vi "updateTriggerList.vi"(8 "error in (no error)":errorcluster, 10 "Trigger list":T1(array[cluster]), 11 "Trigger queue in":refnum<queue>) -> (0 "error out":errorcluster, 1 "Trigger available?":bool, 2 "Updated trigger list":T1(array[cluster]), 3 "Trigger queue out":refnum<queue>)   [LabVIEW 2017]
uses:
  Trigger message.ctl
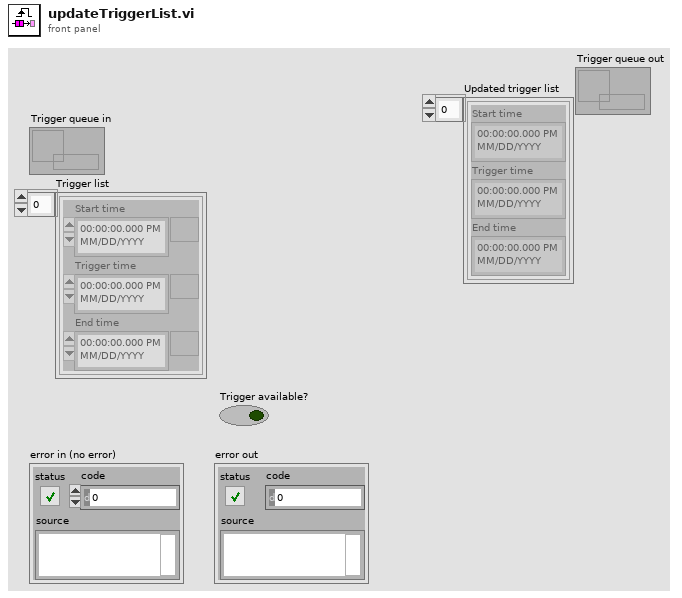
[diagram p1: front panel]
types:
  T1 = cluster{"Start time":timestamp, "Trigger time":timestamp, "End time":timestamp}[]
  T2 = typedef "Trigger message.ctl" = enum16{"New trigger", "Updated trigger"}
  T3 = cluster{"Trigger timestamps":cluster{"Start time":timestamp, "Trigger time":timestamp, "End time":timestamp}, "Message type":T2}
  T4 = cluster{"Start time":timestamp, "Trigger time":timestamp, "End time":timestamp}
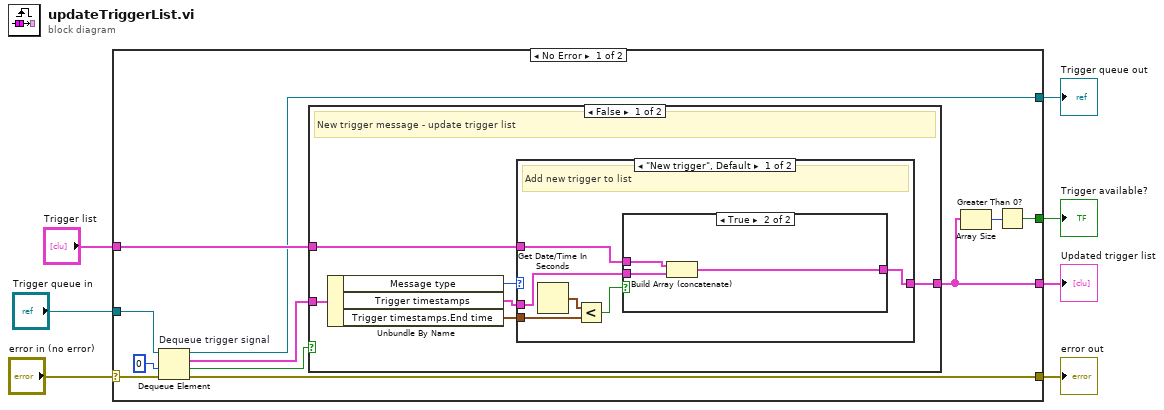
[diagram p0: block diagram]
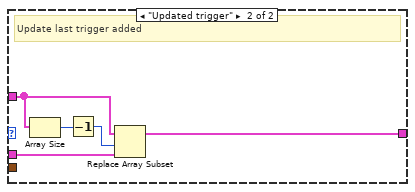
[diagram p3: hidden frame]
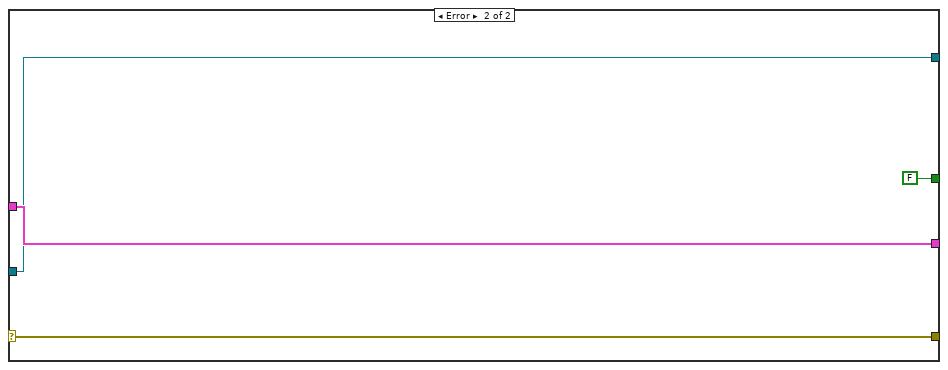
[diagram p5: hidden frame]
diagram:
  n1 = case shown="No Error" "error in (no error)" {
    selector: "error in (no error)" -> [w17 w44]
    tunnel: [w12 w44] -> w7
    tunnel: "Trigger queue in" -> [w16 w42]
    tunnel: "Trigger list" -> [w13 w43]
    tunnel: [w10 w43] -> w3
    tunnel: [w11 w42] -> w2
    tunnel: [w8 FALSE] -> w1
    frame No Error {
      n2 = Dequeue Element "Dequeue trigger signal"(queue=w16, timeout in ms (-1)=0, error in (no error)=w17) -> (queue out=w11:refnum<queue>, element=w14:T3, timed out?=w15:bool, error out=w12:errorcluster)
      n3 = case shown="False" w15 {
        tunnel: w14 -> [w23 _]
        tunnel: w13 -> [w24 w40]
        tunnel: [w20 w40] -> w10
        frame False {
          # "New trigger message - update trigger list"
          n4 = Unbundle By Name(w23) -> ("Message type"=w22:T2, "Trigger timestamps"=w21:T4, "Trigger timestamps.End time"=w19:timestamp)
          n5 = case shown="\"New trigger\", Default" w22 {
            tunnel: w24 -> [w30 w38]
            tunnel: w21 -> [w29 w39]
            tunnel: [w28 w35] -> w20
            tunnel: w19 -> [w25 _]
            frame "New trigger", Default {
              # "Add new trigger to list"
              n6 = Get Date/Time In Seconds() -> (seconds since 1Jan1904=w26:timestamp)
              n7 = Less?(x=w26, y=w25) -> (x < y?=w27:bool)
              n8 = case shown="True" w27 {
                tunnel: w30 -> [w31 w34]
                tunnel: w29 -> [_ w33]
                tunnel: [w31 w32] -> w28
                frame False {
                  # "Trigger period is already over, discard it."
                }
                frame True {
                  n9 = Build Array (concatenate)(w34, w33) -> (w32:T1)
                }
              }
            }
            frame "Updated trigger" {
              # "Update last trigger added"
              n10 = Array Size(array=w38) -> (size(s)=w37:i32)
              n11 = Decrement(x=w37) -> (x-1=w36:i32)
              n12 = Replace Array Subset(array=w38, new element=w39, index=w36) -> (w35:T1)
            }
          }
        }
        frame True {
          # "No new trigger"
        }
      }
      n13 = Array Size(array=w10) -> (size(s)=w9:i32)
      n14 = Greater Than 0?(x=w9) -> (x > 0?=w8:bool)
    }
    frame Error {
    }
  }
  "error out" <- w7
  "Updated trigger list" <- w3
  "Trigger queue out" <- w2
  "Trigger available?" <- w1
